vi "Get Data Channels.vi"(0 "Timed Node in":refnum<class "AMS Climate Chamber Template.lvclass">, 5 "error in":errorcluster) -> (14 "Timed Node out":refnum<class "AMS Climate Chamber Template.lvclass">, 15 "FIFO Consumer Channels":string[][](array[string]), 16 "Tag Consumer Channels":string[][](array[string]), 17 "FIFO Producer Channels":string[][](array[string]), 18 "Tag Producer Channels":string[][](array[string]), 19 "error out":errorcluster)   [LabVIEW 2023, in "AMS Climate Chamber Template.lvlib" / "AMS Climate Chamber Template.lvclass"]
uses:
  AMS Climate Chamber Template.lvclass
  <vilib>/ADAS Replay HIL/Template Node/Plugin/Template Node/Template Node.lvclass
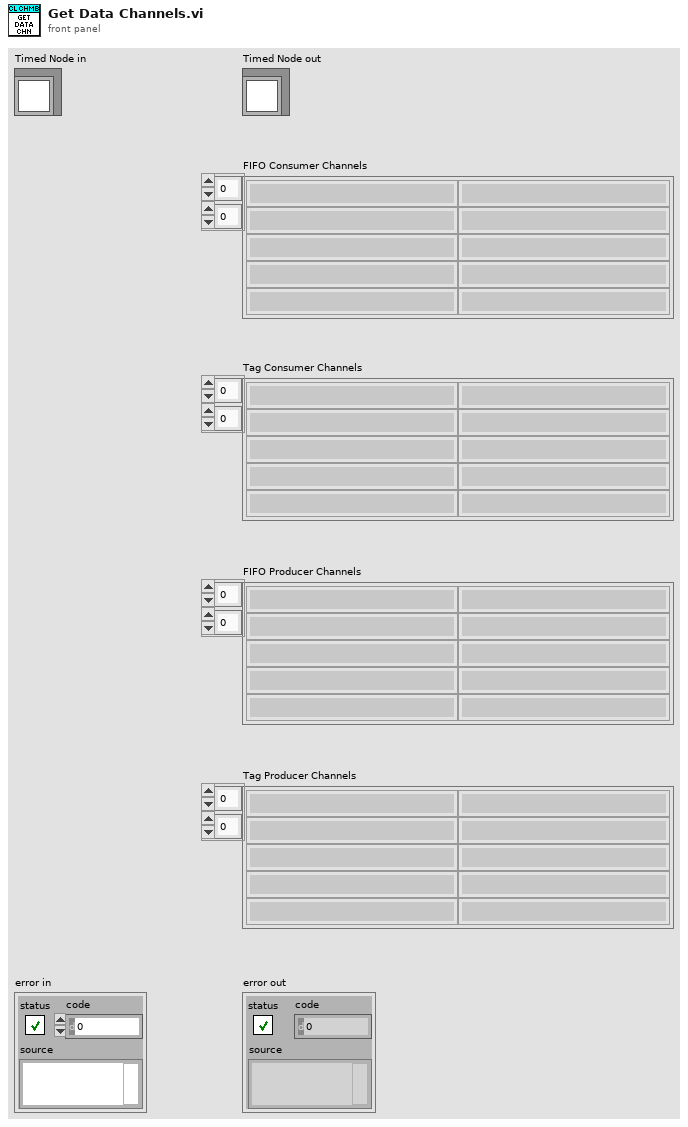
[diagram p1: front panel]
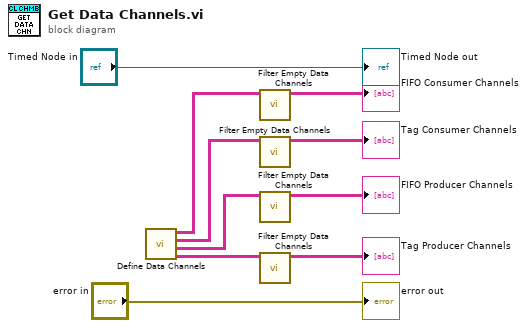
[diagram p0: block diagram]
diagram:
  n1 = call "Define Data Channels.vi"() -> ("Tag Producer Channels"=w6:string[][], "FIFO Producer Channels"=w7:string[][], "Tag Consumer Channels"=w8:string[][], "FIFO Consumer Channels"=w5:string[][])  [unwired: 8 in]
  n2 = call <vilib>:"Filter Empty Data Channels.vi"("Data Channels in"=w5) -> ("Data Channels out"=→"FIFO Consumer Channels":string[][])  [unwired: 10 in]
  n3 = call <vilib>:"Filter Empty Data Channels.vi"("Data Channels in"=w8) -> ("Data Channels out"=→"Tag Consumer Channels":string[][])  [unwired: 10 in]
  n4 = call <vilib>:"Filter Empty Data Channels.vi"("Data Channels in"=w7) -> ("Data Channels out"=→"FIFO Producer Channels":string[][])  [unwired: 10 in]
  n5 = call <vilib>:"Filter Empty Data Channels.vi"("Data Channels in"=w6) -> ("Data Channels out"=→"Tag Producer Channels":string[][])  [unwired: 10 in]
  "error out" <- "error in"
  "Timed Node out" <- "Timed Node in"
